vi "prepareCamera.vi"(8 "error in (no error)":errorcluster) -> (0 "error out":errorcluster)   [LabVIEW 2013]
uses:
  Camera/lib/atmcd32d.llb/EMGainMode_mode typedef.ctl
  Camera/lib/atmcd32d.llb/OutputAmplifier_type typedef.ctl
  Camera/lib/atmcd32d.llb/Error Code Enum typedef.ctl
  Camera/lib/atmcd32d.llb/Spool_method typedef.ctl
  Camera/lib/atmcd32d.llb/Shutter_mode typedef.ctl
  Camera/lib/atmcd32d.llb/Shutter_type typedef.ctl
  Camera/lib/atmcd32d.llb/ReadMode_mode typedef.ctl
  Camera/lib/atmcd32d.llb/AcquisitionMode_mode typedef.ctl
  Camera/lib/atmcd32d.llb/TriggerMode_mode typedef.ctl
  Variables/GlobalSetGetConfigureCamera.vi
  Variables/ccdChipPixels.vi
  Variables/GlobalDevice.vi
  Variables/MesaurementModus.vi
  Variables/GlobalGetTimingsFromCamera.vi
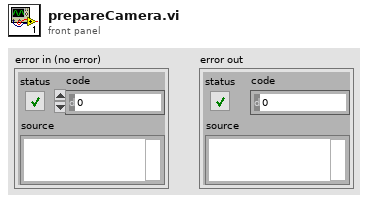
[diagram p1: front panel]
types:
  T1 = typedef "ReadMode_mode typedef.ctl" = enum16{"Full Vertical Binning", "Multi-Track", "Random-Track", "Single-Track", "Image"}
  T2 = typedef "Shutter_type typedef.ctl" = enum16{"TTL Low", "TTL High"}
  T3 = typedef "Shutter_mode typedef.ctl" = enum16{"Auto", "Open", "Close"}
  T4 = typedef "Spool_method typedef.ctl" = enum16{"32-bit", "Depends", "16-bit", "Multiple Directory", "Spool to RAM disk", "16-bit FITS", "SIF", "16-buit TIFF", "Multiple Directory Compressed"}
  T5 = typedef "Error Code Enum typedef.ctl" = enum32{"N/A (0)", "DRV_ERROR_CODES", "DRV_SUCCESS", "DRV_VXDNOTINSTALLED", "DRV_ERROR_SCAN", "DRV_ERROR_CHECK_SUM", "DRV_ERROR_FILELOAD", "DRV_UNKNOWN_FUNC", "DRV_ERROR_VXD_INIT", "DRV_ERROR_ADDRESS", "DRV_ERROR_PAGELOCK", "DRV_ERROR_PAGEUNLOCK", "DRV_ERROR_BOARDTEST", "DRV_ERROR_ACK", "DRV_ERROR_UP_FIFO", "DRV_ERROR_PATTERN", "N/A (16)", "DRV_ACQUISITION_ERRORS", "DRV_ACQ_BUFFER", "DRV_ACQ_DOWNFIFO_FULL", "DRV_PROC_UNKONWN_INSTRUCTION", "DRV_ILLEGAL_OP_CODE", "DRV_KINETIC_TIME_NOT_MET", "DRV_ACCUM_TIME_NOT_MET", "DRV_NO_NEW_DATA", "N/A (25)", "DRV_SPOOLERROR", "N/A (27)", "N/A (28)", "N/A (29)", "N/A (30)", "N/A (31)", "N/A (32)", "DRV_TEMPERATURE_CODES", "DRV_TEMPERATURE_OFF", "DRV_TEMPERATURE_NOT_STABILIZED", "DRV_TEMPERATURE_STABILIZED", "DRV_TEMPERATURE_NOT_REACHED", "DRV_TEMPERATURE_OUT_RANGE", "DRV_TEMPERATURE_NOT_SUPPORTED", "DRV_TEMPERATURE_DRIFT", "N/A (41)", "N/A (42)", "N/A (43)", "N/A (44)", "N/A (45)", "N/A (46)", "N/A (47)", "N/A (48)", "DRV_GENERAL_ERRORS", "DRV_INVALID_AUX", "DRV_COF_NOTLOADED", "DRV_FPGAPROG", "DRV_FLEXERROR", "DRV_GPIBERROR", "N/A (55)", "N/A (56)", "N/A (57)", "N/A (58)", "N/A (59)", "N/A (60)", "N/A (61)", "N/A (62)", "N/A (63)", "DRV_DATATYPE", "DRV_DRIVER_ERRORS", "DRV_P1INVALID", "DRV_P2INVALID", "DRV_P3INVALID", "DRV_P4INVALID", "DRV_INIERROR", "DRV_COFERROR", "DRV_ACQUIRING", "DRV_IDLE", "DRV_TEMPCYCLE", "DRV_NOT_INITIALIZED", "DRV_P5INVALID", "DRV_P6INVALID", "DRV_INVALID_MODE", "DRV_INVALID_FILTER", "DRV_I2CERRORS", "DRV_I2CDEVNOTFOUND", "DRV_I2CTIMEOUT", "DRV_P7INVALID", "N/A (84)", "N/A (85)", "N/A (86)", "N/A (87)", "N/A (88)", "N/A (89)", "DRV_IOCERROR", "DRV_VRMVERSIONERROR"}
  T6 = typedef "OutputAmplifier_type typedef.ctl" = enum16{"Standard EMCCD gain register", "Conventional CCD register"}
  T7 = typedef "EMGainMode_mode typedef.ctl" = enum16{"8-bit", "12-bit", "Linear", "Real"}
  T8 = typedef "TriggerMode_mode typedef.ctl" = enum16{"Internal", "External", "N/A (2)", "N/A (3)", "N/A (4)", "N/A (5)", "External Start"}
  T9 = typedef "AcquisitionMode_mode typedef.ctl" = enum16{"Reserved (0)", "Single Scan", "Accumulate", "Kinetics", "Fast Kinetics", "Run Till Abort", "Reserved (6)", "Reserved (7)", "Reserved (8)", "Time Delayed Integration"}
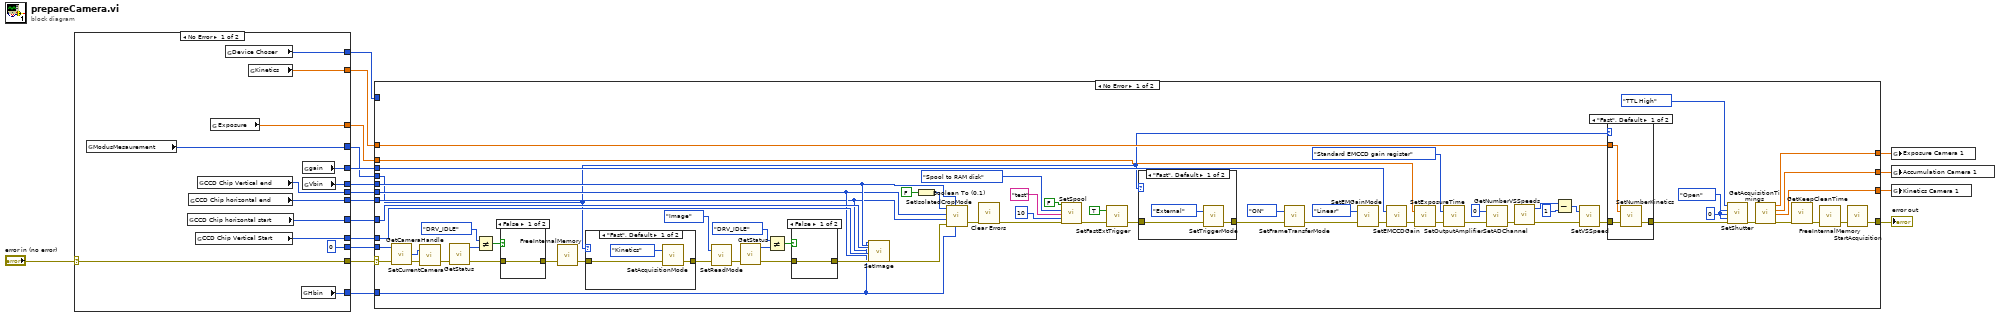
[diagram p0: block diagram]
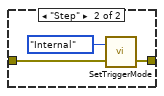
[diagram p4: hidden frame]
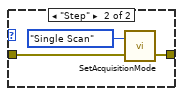
[diagram p5: hidden frame]
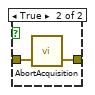
[diagram p6: hidden frame]
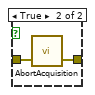
[diagram p7: hidden frame]
diagram:
  n1 = case shown="No Error" "error in (no error)" {
    selector: "error in (no error)" -> [w23 _]
    tunnel: [w31 _] -> w3
    tunnel: [w30 _] -> w4
    tunnel: [w29 _] -> w5
    tunnel: [w28 _] -> w6
    tunnel: [0 ("camerahandler") _] -> w8
    tunnel: [w27 _] -> w9
    tunnel: [w26 _] -> w10
    tunnel: [w25 _] -> w13
    tunnel: [w24 _] -> w14
    tunnel: [w23 _] -> w12
    tunnel: [w21 _] -> w15
    tunnel: [w19 _] -> w2
    tunnel: [w20 _] -> w1
    frame No Error {
      n2 = global read "MesaurementModus.vi" "ModusMesaurement"() -> (w20:enum32{"Fast", "Step"})
      n3 = global read "ccdChipPixels.vi" "CCD Chip horizontal start"() -> (w27:i32)
      n4 = global read "ccdChipPixels.vi" "CCD Chip horizontal end"() -> (w25:i32)
      n5 = global read "ccdChipPixels.vi" "CCD Chip Vertical Start"() -> (w26:i32)
      n6 = global read "ccdChipPixels.vi" "CCD Chip Vertical end"() -> (w24:i32)
      n7 = global read "GlobalSetGetConfigureCamera.vi" "Exposure"() -> (w31:sgl)
      n8 = global read "GlobalDevice.vi" "Device Choser"() -> (w21:enum32{"Stage", "Mirror"})
      n9 = global read "GlobalSetGetConfigureCamera.vi" "Kinetics"() -> (w19:sgl)
      n10 = global read "GlobalSetGetConfigureCamera.vi" "Hbin"() -> (w29:i32)
      n11 = global read "GlobalSetGetConfigureCamera.vi" "gain"() -> (w28:i32)
      n12 = global read "GlobalSetGetConfigureCamera.vi" "Vbin"() -> (w30:i32)
    }
    frame Error {
    }
  }
  n13 = case shown="No Error" w12 {
    selector: w12 -> [w67 _]
    tunnel: w3 -> [w99 _]
    tunnel: [w100 _] -> w18
    tunnel: w5 -> [w55 _]
    tunnel: w4 -> [w56 _]
    tunnel: [w72 _] -> w17
    tunnel: w6 -> [w98 _]
    tunnel: [w71 _] -> w7
    tunnel: w8 -> [w70 _]
    tunnel: w9 -> [w69 _]
    tunnel: w10 -> [w68 _]
    tunnel: [w57 _] -> w16
    tunnel: w13 -> [w48 _]
    tunnel: w14 -> [w49 _]
    tunnel: w15 -> [_ _]
    tunnel: w2 -> [w34 _]
    tunnel: w1 -> [w32 _]
    frame No Error {
      w41 = 0 ("closingtime")
      n14 = call "GetCameraHandle.vi"("error in (no error)"=w67, "cameraIndex"=w70) -> ("error out"=w96:errorcluster, "cameraHandle"=w97:i32)  [unwired: 1 in, 1 out]
      n15 = call "SetCurrentCamera.vi"("error in (no error)"=w96, "cameraHandle"=w97) -> ("error out"=w95:errorcluster)  [unwired: 1 out]
      n16 = call "GetStatus.vi"("error in (no error)"=w95) -> ("error out"=w33:errorcluster, "status"=w93:T5)  [unwired: 2 in, 1 out]
      n17 = Not Equal?(x=Error_Code_Enum_typedef."DRV_IDLE" ("status"), y=w93) -> (x != y?=w92:bool)
      n18 = case shown="False" w92 {
        tunnel: w33 -> [w120 w122]
        tunnel: [w120 w121] -> w39
        frame False {
        }
        frame True {
          n19 = call "AbortAcquisition.vi"("error in (no error)"=w122) -> ("error out"=w121:errorcluster)  [unwired: 1 in, 1 out]
        }
      }
      n20 = call "FreeInternalMemory.vi"("error in (no error)"=w39) -> ("error out"=w58:errorcluster)  [unwired: 1 in, 1 out]
      n21 = case shown="\"Fast\", Default" w32 {
        tunnel: w58 -> [w113 w115]
        tunnel: [w112 w116] -> w35
        frame "Fast", Default {
          n22 = call "SetAcquisitionMode.vi"("error in (no error)"=w113, "mode"=AcquisitionMode_mode_typedef."Kinetics") -> ("error out"=w112:errorcluster)  [unwired: 1 out]
        }
        frame "Step" {
          n23 = call "SetAcquisitionMode.vi"("error in (no error)"=w115, "mode"=AcquisitionMode_mode_typedef."Single Scan") -> ("error out"=w116:errorcluster)  [unwired: 1 out]
        }
      }
      n24 = call "SetReadMode.vi"("error in (no error)"=w35, "mode"=ReadMode_mode_typedef."Image") -> ("error out"=w60:errorcluster)  [unwired: 1 out]
      n25 = call "GetStatus.vi"("error in (no error)"=w60) -> ("error out"=w61:errorcluster, "status"=w63:T5)  [unwired: 2 in, 1 out]
      n26 = Not Equal?(x=Error_Code_Enum_typedef."DRV_IDLE" ("status"), y=w63) -> (x != y?=w62:bool)
      n27 = case shown="False" w62 {
        tunnel: w61 -> [w117 w119]
        tunnel: [w117 w118] -> w59
        frame False {
        }
        frame True {
          n28 = call "AbortAcquisition.vi"("error in (no error)"=w119) -> ("error out"=w118:errorcluster)  [unwired: 1 in, 1 out]
        }
      }
      n29 = call "SetImage.vi"("hbin"=w55, "vbin"=w56, "hstart"=w69, "hend"=w48, "vstart"=w68, "vend"=w49, "error in (no error)"=w59) -> ("error out"=w50:errorcluster)  [unwired: 19 in, 1 out]
      n30 = Boolean To (0,1)(Boolean=FALSE) -> (0, 1=w46:i16)
      n31 = call "SetIsolatedCropMode.vi"("hbin"=w55, "vbin"=w56, "error in (no error)"=w50, "cropWidth"=w48, "cropHeight"=w49, "active"=w46) -> ("error out"=w45:errorcluster)  [unwired: 1 out]
      n32 = call <vilib>:"Clear Errors.vi"("error in (no error)"=w45) -> ("error out"=w44:errorcluster)  [unwired: 6 in]
      n33 = call "SetSpool.vi"("active"=FALSE, "method"=Spool_method_typedef."Spool to RAM disk", "name"="test", "framebuffersize (10)"=10, "error in (no error)"=w44) -> ("error out"=w43:errorcluster)  [unwired: 9 in, 1 out]
      n34 = call "SetFastExtTrigger.vi"("error in (no error)"=w43, "mode"=TRUE) -> ("error out"=w37:errorcluster)  [unwired: 1 out]
      n35 = case shown="\"Fast\", Default" w32 {
        tunnel: [w107 w110] -> w90
        tunnel: w37 -> [w105 w109]
        frame "Fast", Default {
          n36 = call "SetTriggerMode.vi"("error in (no error)"=w105, "mode"=TriggerMode_mode_typedef."External") -> ("error out"=w107:errorcluster)  [unwired: 1 out]
        }
        frame "Step" {
          n37 = call "SetTriggerMode.vi"("error in (no error)"=w109, "mode"=TriggerMode_mode_typedef."Internal") -> ("error out"=w110:errorcluster)  [unwired: 1 out]
        }
      }
      n38 = call "SetFrameTransferMode.vi"("error in (no error)"=w90, "mode"=enum16{"OFF", "ON"}."ON") -> ("error out"=w73:errorcluster)  [unwired: 1 out]
      n39 = call "SetEMGainMode.vi"("error in (no error)"=w73, "mode"=EMGainMode_mode_typedef."Linear") -> ("error out"=w78:errorcluster)  [unwired: 1 out]
      n40 = call "SetEMCCDGain.vi"("error in (no error)"=w78, "gain"=w98) -> ("error out"=w77:errorcluster)  [unwired: 1 out]
      n41 = call "SetExposureTime.vi"("error in (no error)"=w77, "time"=w99) -> ("error out"=w76:errorcluster)  [unwired: 1 out]
      n42 = call "SetOutputAmplifier.vi"("error in (no error)"=w76, "type"=OutputAmplifier_type_typedef."Standard EMCCD gain register") -> ("error out"=w75:errorcluster)  [unwired: 1 out]
      n43 = call "SetADChannel.vi"("error in (no error)"=w75, "channel"=0) -> ("error out"=w88:errorcluster)  [unwired: 1 out]
      n44 = call "GetNumberVSSpeeds.vi"("error in (no error)"=w88) -> ("error out"=w87:errorcluster, "number"=w86:i32)  [unwired: 2 in, 1 out]
      n45 = Subtract(x=w86, y=1) -> (x-y=w84:i32)
      n46 = call "SetVSSpeed.vi"("error in (no error)"=w87, "index"=w84) -> ("error out"=w83:errorcluster)  [unwired: 1 out]
      n47 = case shown="\"Fast\", Default" w32 {
        tunnel: w83 -> [w103 w104]
        tunnel: [w102 w104] -> w82
        tunnel: w34 -> [w101 _]
        frame "Fast", Default {
          n48 = call "SetNumberKinetics.vi"("error in (no error)"=w103, "number"=w101) -> ("error out"=w102:errorcluster)  [unwired: 1 out]
        }
        frame "Step" {
        }
      }
      n49 = call "SetShutter.vi"("type"=Shutter_type_typedef."TTL High", "mode"=Shutter_mode_typedef."Open", "closingtime"=w41, "openingtime"=w41, "error in (no error)"=w82) -> ("error out"=w81:errorcluster)  [unwired: 9 in, 1 out]
      n50 = call "GetAcquisitionTimings.vi"("error in (no error)"=w81) -> ("exposure"=w57:sgl, "accumulate"=w71:sgl, "kinetic"=w72:sgl, "error out"=w80:errorcluster)  [unwired: 10 in, 1 out]
      n51 = call "GetKeepCleanTime.vi"("error in (no error)"=w80) -> ("error out"=w66:errorcluster)  [unwired: 4 in, 2 out]
      n52 = call "FreeInternalMemory.vi"("error in (no error)"=w66) -> ("error out"=w65:errorcluster)  [unwired: 1 in, 1 out]
      n53 = call "StartAcquisition.vi"("error in (no error)"=w65) -> ("error out"=w100:errorcluster)  [unwired: 1 in, 1 out]
    }
    frame Error {
    }
  }
  "error out" <- w18
  n54 = global write "GlobalGetTimingsFromCamera.vi" "Exposure Camera 1"(w16) -> ()
  n55 = global write "GlobalGetTimingsFromCamera.vi" "Accumulation Camera 1"(w7) -> ()
  n56 = global write "GlobalGetTimingsFromCamera.vi" "Kinetics Camera 1"(w17) -> ()
